vi "MovCor-QueueStartStop.vi"(8 "error in (no error)":errorcluster, 9 "Next START State (None)":T1, 10 "Main prrotocol Starting/Stopped":T2, 11 "UI queue in":refnum<queue>) -> (0 "error out":errorcluster, 3 "UI queue out":refnum<queue>)   [LabVIEW 2020]
uses:
  Queue/Message Queue/Typedefs/Message Cluster.ctl
  Typedefs/Start-Stop Enum.ctl
  Typedefs/Top level VI states.ctl
  Typedefs/HW config states enum.ctl
  Global Variables/General Globals.vi
panel:
  # "<--- Wire only when \"Main prrotocol Starting/Stopped\" is \"START\""
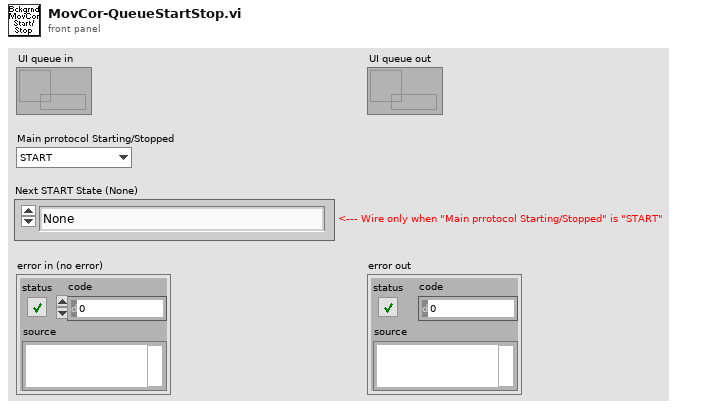
[diagram p1: front panel]
types:
  T1 = typedef "Top level VI states.ctl" = enum16{"None", "Initialise UI", "<STACK PROTOCOL STATES>", "AOL Zstack-START", "AOL Zstack-STOP", "Motor Zstack-START", "Motor Zstack-STOP", "<ACQUISITION PROTOCOL STATES> ", "Functional Acquisition-START", "Functional Acquisition-STOP", "Single Plane Acquisition-START", "Single Plane Acquisition-STOP", "Volume Acquisition-START", "Volume Acquisition-STOP", "<LIVE IMAGING PROTOCOL STATES>", "Live Imaging-START", "Live Imaging-STOP", "Live Plane Imaging-START", "Live Plane Imaging-STOP", "Live Volume Imaging-START", "Live Volume Imaging-STOP", "<MOVEMENT CORRECTION PROTOCOL STATES>", "EXIT"}
  T2 = typedef "Start-Stop Enum.ctl" = enum16{"START", "STOP"}
  T3 = typedef "HW config states enum.ctl" = enum16{"Load from file", "Save to file", "Save backup", "Write all", "Read all", "Write XY stage settings", "Write DAQ FPGA settings", "Write Control FPGA settings", "Write Phys Channels", "Write System Config", "Write HW Config", "Save System Config", "Save HW Config", "Clear", "Compare from file"}
  T4 = typedef "Hardware Configuration settings.ctl" = cluster{"Dev. PC":bool, "Swap XY on stage":bool, "No of AOD":u8, "MC Supported":bool, "Axial MC":bool, "Computer MAC address":string, "Externalise Triggers":bool, "Trigger HW config":T5, "DAQmx Chan":T6, "XY stage available":bool, "XY Stage":T7, "Z stage available":bool, "Z Stage config cluster":T8, "Encoder available":bool, "Encoder":T9, "VidRec available":bool, "Cam VidRec":T10, "Laser Power Control HW config":T11, "Laser 1 available":bool, "Laser 1 config cluster":T12, "Prechirper 1 available":bool, "Prechirper 1 config cluster":T13, "Control system.FPGA available?":bool, "Control Sys. HW config":T14, "DAQ FPGA HW Config":T15, "PMT Voltage Range":T19}
  T5 = typedef "Triggers HW config.ctl" = cluster{"Available Device List":i32, "Device Address":string}
  T6 = typedef "DAQmx physical channels cluster.ctl" = cluster{"Pockels AO":tag, "Hard shutter AO":tag, "PMT AOs":tag, "Galvo AOs":tag, "Power meter AI":tag}
  T7 = typedef "XY Stage config cluster.ctl" = cluster{"COM port":refnum<visa-resource-name>, "Baudrate":i32, "Type":string}
  T8 = typedef "Z Stage config cluster.ctl" = cluster{"COM port":refnum<visa-resource-name>, "Baudrate":i32, "Type":string}
  T9 = typedef "Encoder config cluster.ctl" = cluster{"IP address":string, "Port":u16, "Wheel radius (cm)":dbl, "Encoder Trigger":tag}
  T10 = typedef "Cam VidRec HW config setup cluster.ctl" = cluster{"DO flag-Video record":tag, "DO flag-Trial start":tag}
  T11 = typedef "Laser Power Control HW config.ctl" = cluster{"Laser Power Control":string, "Laser Power Modulation Control":enum16{"NI", "FPGA"}}
  T12 = typedef "Laser 1 config cluster.ctl" = cluster{"COM port":refnum<visa-resource-name>, "Baud Rate":i32, "Type":string}
  T13 = typedef "PreChirper 1 config cluster.ctl" = cluster{"Type":string, "Baud Rate":i32, "COM port":refnum<visa-resource-name>}
  T14 = typedef "Control Sys HW config cluster.ctl" = cluster{"Control system.FPGA Type":enum16{"Virtex 5", "Virtex 7"}, "Control system.Network adapter name":string, "Control system.MAC address":string, "Control system.Ethernet Port":u32, "Control system.Ethernet Port Opened":bool}
  T15 = typedef "DAQ FPGA HW config cluster.ctl" = cluster{"FGPA Ref":T16, "Target":T17, "input card type":T18}
  T16 = typedef "FPGA Ref.ctl" = refnum<k20>
  T17 = typedef "nirio_resource_hc.ctl" = tag
  T18 = typedef "FPGA input type AC-DC.ctl" = enum16{"AC Card", "DC Card"}
  T19 = typedef "PMT Voltage Range.ctl" = cluster{"PMT Voltage Lower Limit":dbl, "PMT Voltage Upper Limit":dbl}
  T20 = typedef "Top level VI states.ctl" = enum16{"None", "Initialise UI", "<STACK PROTOCOL STATES>", "AOL Zstack-START", "AOL Zstack-STOP", "Motor Zstack-START", "Motor Zstack-STOP", "<ACQUISITION PROTOCOL STATES> ", "Functional Acquisition-START", "Functional Acquisition-STOP", "Single Plane Acquisition-START", "Single Plane Acquisition-STOP", "Volume Acquisition-START", "Volume Acquisition-STOP", "<LIVE IMAGING PROTOCOL STATES>", "Live Imaging-START", "Live Imaging-STOP", "Live Plane Imaging-START", "Live Plane Imaging-STOP", "Live Volume Imaging-START", "Live Volume Imaging-STOP", "<MOVEMENT CORRECTION PROTOCOL STATES>", "Background MovCor-START", "Background MovCor-STOP", "EXIT"}
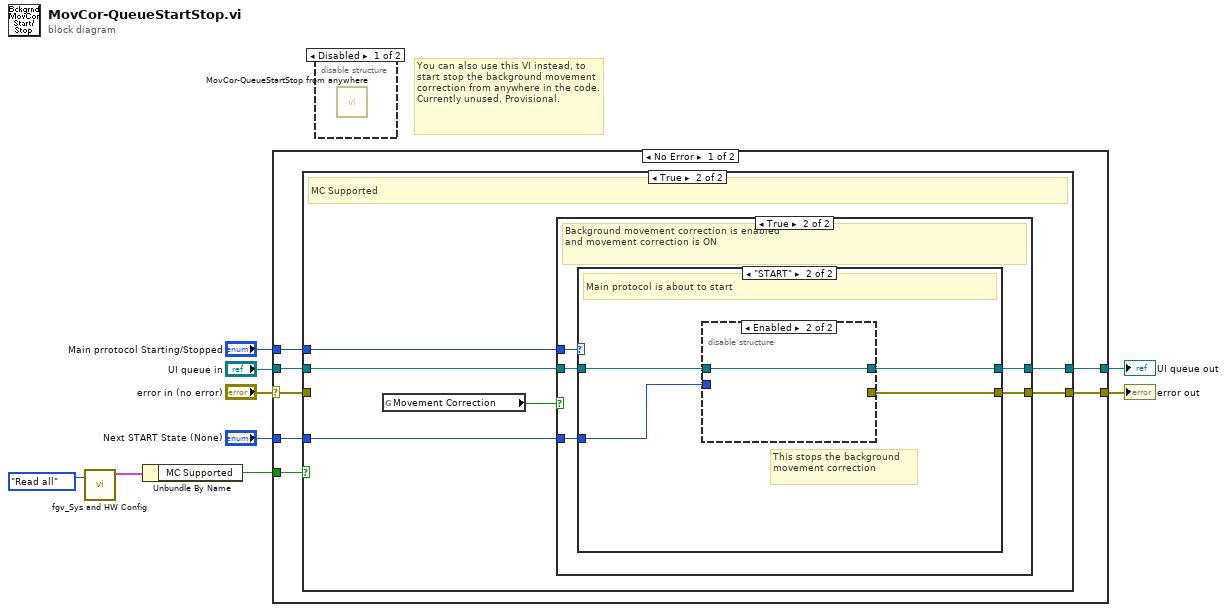
[diagram p0: block diagram]
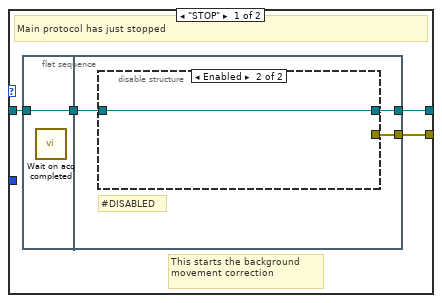
[diagram p5: hidden frame]
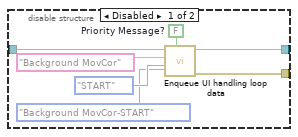
[diagram p6: hidden frame]
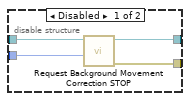
[diagram p7: hidden frame]
diagram:
  # "You can also use this VI instead, to start stop the background movement correction from anywhere in the code. Currently unused. Provisional."
  n1 = call "fgv_Sys and HW Config.vi"("Function"=HW_config_states_enum."Read all") -> ("Hardware Configuration OUT"=w2:T4)  [unwired: 8 in, 2 out]
  n2 = Unbundle By Name(w2) -> ("MC Supported"=w1:bool)
  n3 = case shown="No Error" "error in (no error)" {
    selector: "error in (no error)" -> [w11 w56]
    tunnel: "Main prrotocol Starting/Stopped" -> [w16 _]
    tunnel: "UI queue in" -> [w15 w57]
    tunnel: [w14 w56] -> w8
    tunnel: [w13 w57] -> w9
    tunnel: "Next START State (None)" -> [w12 _]
    tunnel: w1 -> [w10 _]
    frame No Error {
      n4 = case shown="True" w10 {
        tunnel: w16 -> [_ w24]
        tunnel: w15 -> [w18 w23]
        tunnel: [w17 w22] -> w14
        tunnel: [w18 w21] -> w13
        tunnel: w12 -> [_ w20]
        tunnel: w11 -> [w17 _]
        frame False {
          # "MovCor Unsupported"
        }
        frame True {
          # "MC Supported"
          n5 = global read "General Globals.vi" "Movement Correction"() -> (w19:bool)
          n6 = case shown="True" w19 {
            tunnel: w23 -> [w25 w30]
            tunnel: [_ w29] -> w22
            tunnel: w24 -> [_ w27]
            tunnel: [w25 w28] -> w21
            tunnel: w20 -> [_ w26]
            frame False {
              # "Background movement correction is disabled\nor movement correction is OFF"
            }
            frame True {
              # "Background movement correction is enabled\nand movement correction is ON"
              n7 = case shown="\"START\"" w27 {
                tunnel: w30 -> [w34 w50]
                tunnel: [w33 w49] -> w29
                tunnel: [w32 w48] -> w28
                tunnel: w26 -> [_ w47]
                frame "STOP" {
                  # "This starts the background movement correction"
                  # "Main protocol has just stopped"
                  n8 = flat-sequence {
                    tunnel: w34 -> [w35]
                    tunnel: [w35] -> w31
                    tunnel: [w37] -> w33
                    tunnel: [w36] -> w32
                    tunnel: w31 -> [w38]
                    frame #0 {
                      n9 = call "Wait on acq completed.vi"() -> ()  [unwired: 11 in, 1 out]
                    }
                    frame #1 {
                      # "#DISABLED"
                      n10 = disable-structure shown="Enabled" {
                        disable-tunnel: w38 -> [w44 w46]
                        disable-tunnel: [w43 _] -> w37
                        disable-tunnel: [w41 w46] -> w36
                        frame Disabled {
                          w39 = FALSE  # Priority Message?
                          n11 = call "Enqueue UI handling loop data.vi"("Next State"=Top_level_VI_states."Background MovCor-START", "Priority Message? (T)"=w39, "Start/Stop"=Start-Stop_Enum."START", "Message"="Background MovCor", "Queue in"=w44) -> ("error out"=w43:errorcluster, "Queue out"=w41:refnum<queue>)  [unwired: 5 in]
                        }
                        frame Enabled {
                        }
                      }
                    }
                  }
                }
                frame "START" {
                  # "This stops the background movement correction"
                  # "Main protocol is about to start"
                  n12 = disable-structure shown="Enabled" {
                    disable-tunnel: w50 -> [w54 w55]
                    disable-tunnel: [w53 _] -> w49
                    disable-tunnel: [w52 w55] -> w48
                    disable-tunnel: w47 -> [w51 _]
                    frame Disabled {
                      n13 = call "Request Background Movement Correction STOP.vi"("Next State"=w51, "UI queue in"=w54) -> ("error out"=w53:errorcluster, "UI queue out"=w52:refnum<queue>)  [unwired: 8 in]
                    }
                    frame Enabled {
                    }
                  }
                }
              }
            }
          }
        }
      }
    }
    frame Error {
    }
  }
  "error out" <- w8
  "UI queue out" <- w9
  n14 = disable-structure shown="Disabled" {
    frame Disabled {
      n15 = call "MovCor-QueueStartStop from anywhere.vi"() -> ()  [unwired: 11 in, 1 out]
    }
    frame Enabled {
    }
  }
